vi "ReadWait.vi"(8 "error in (no error)":errorcluster, 9 "Value":bool=TRUE, 10 "Read":i32, 11 "I-O in":refnum<class "I-O.lvclass">) -> (0 "error out":errorcluster, 3 "I-O out":refnum<class "I-O.lvclass">)   [LabVIEW 2020, in "I-O.lvclass"]
uses:
  I-O.lvclass
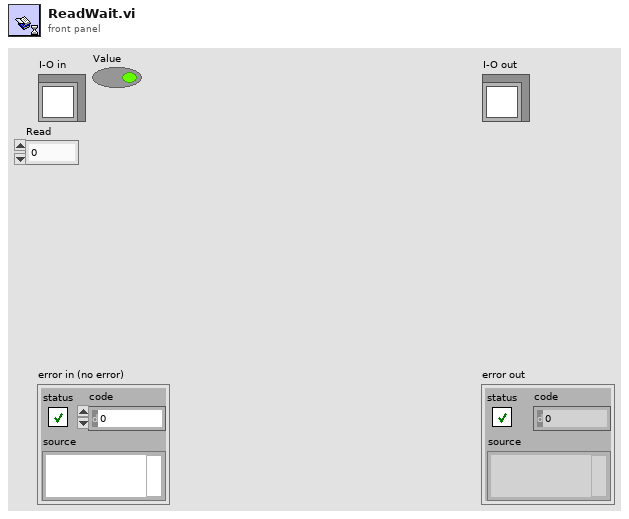
[diagram p1: front panel]
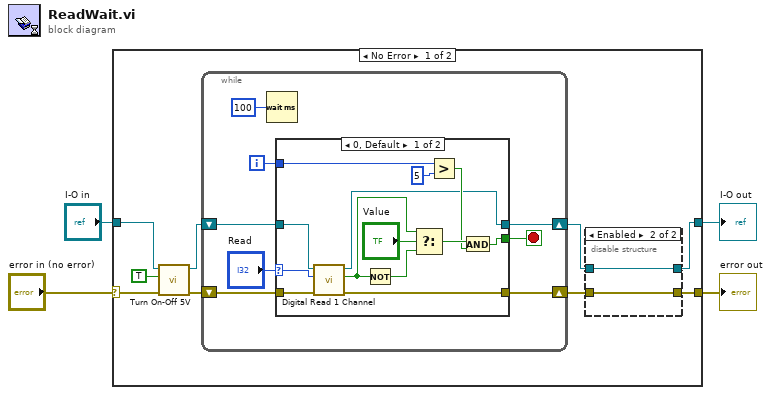
[diagram p0: block diagram]
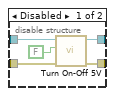
[diagram p2: hidden frame]
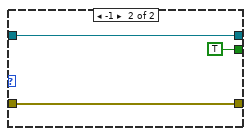
[diagram p3: hidden frame]
diagram:
  n1 = case shown="No Error" "error in (no error)" {
    selector: "error in (no error)" -> [w8 w46]
    tunnel: [w5 w46] -> w3
    tunnel: [w11 w45] -> w1
    tunnel: "I-O in" -> [w12 w45]
    frame No Error {
      n2 = call-dynamic "Turn On-Off 5V.vi"("error in (no error)"=w8, "Value"=TRUE, "I-O in"=w12) -> ("error out"=w7:errorcluster, "I-O out"=w10:refnum<class "I-O.lvclass">)  [unwired: 7 in]
      n3 = while {
        shift-right: [w24] -> w9
        shift-left: w10 -> [w25]
        shift-right: [w22] -> w6
        shift-left: w7 -> [w23]
        i -> [w27]
        stop <- w26 stop-if-true
        n4 = Wait (ms)(milliseconds to wait=u32 100) -> ()  [unwired: 1 out]
        n5 = case shown="0, Default" "Read" {
          selector: "Read" -> [w30 _]
          tunnel: w27 -> [w40 _]
          tunnel: [w36 TRUE] -> w26
          tunnel: w25 -> [w35 w44]
          tunnel: [w33 w44] -> w24
          tunnel: w23 -> [w32 w42]
          tunnel: [w31 w42] -> w22
          frame 0, Default {
            n6 = call-dynamic "Digital Read 1 Channel.vi"("error in (no error)"=w32, "Read"=w30, "I-O in"=w35) -> ("error out"=w31:errorcluster, "Value"=w34:bool, "I-O out"=w33:refnum<class "I-O.lvclass">)  [unwired: 6 in]
            n7 = Not(x=w34) -> (.not. x?=w41:bool)
            n8 = Select(t=w34, s="Value", f=w41) -> (s? t:f=w38:bool)
            n9 = Greater?(x=w40, y=5) -> (0:w37:bool)
            n10 = And(x=w38, y=w37) -> (x .and. y?=w36:bool)
          }
          frame -1 {
          }
        }
      }
      n11 = disable-structure shown="Enabled" {
        disable-tunnel: [w18 w20] -> w11
        disable-tunnel: w9 -> [w17 w20]
        disable-tunnel: w6 -> [w16 w19]
        disable-tunnel: [w15 w19] -> w5
        frame Disabled {
          n12 = call-dynamic "Turn On-Off 5V.vi"("error in (no error)"=w16, "Value"=FALSE, "I-O in"=w17) -> ("error out"=w15:errorcluster, "I-O out"=w18:refnum<class "I-O.lvclass">)  [unwired: 7 in]
        }
        frame Enabled {
        }
      }
    }
    frame Error {
    }
  }
  "error out" <- w3
  "I-O out" <- w1
